vi "Encrypt file path creation.vi"(8 "error in (no error)":errorcluster) -> (0 "error out":errorcluster, 3 "File Path":path)   [LabVIEW 2025]
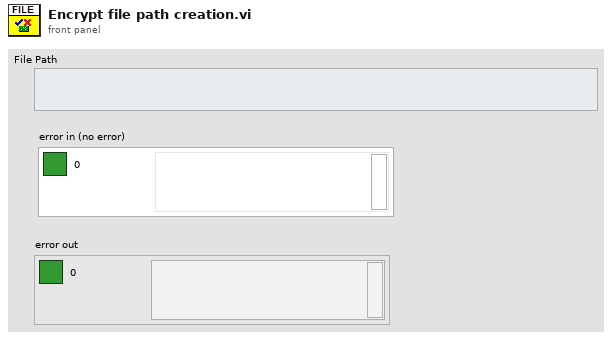
[diagram p1: front panel]
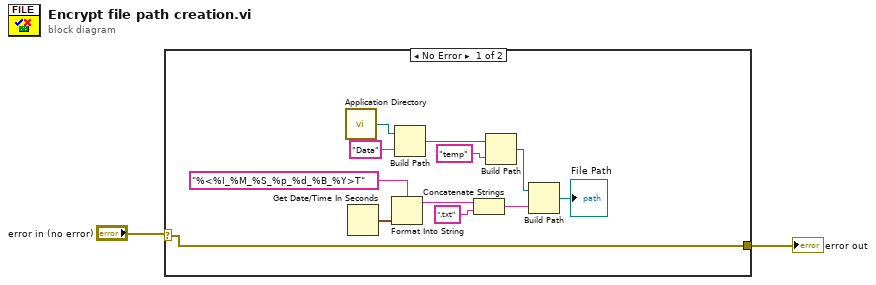
[diagram p0: block diagram]
diagram:
  n1 = case shown="No Error" "error in (no error)" {
    selector: "error in (no error)" -> [w3 _]
    tunnel: [w3 _] -> w1
    frame No Error {
      n2 = call <vilib>:"Application Directory.vi"() -> ("Application Directory"=w14:path)
      n3 = Get Date/Time In Seconds() -> (seconds since 1Jan1904=w9:timestamp)
      n4 = Format Into String(format string="%<%I_%M_%S_%p_%d_%B_%Y>T", w9) -> (resulting string=w8:string)  [unwired: 2 in, 1 out]
      n5 = Build Path(base path=w14, name or relative path="Data") -> (appended path=w12:path)
      n6 = Concatenate Strings(w8, ".txt" ("string")) -> (w5:string)
      n7 = Build Path(base path=w12, name or relative path="temp") -> (appended path=w6:path)
      n8 = Build Path(base path=w6, name or relative path=w5) -> (appended path=→"File Path":path)
    }
    frame Error {
    }
  }
  "error out" <- w1
